vi "Check VIs for Dynamic Call Compatibility.vi"(8 "error in (no error)":errorcluster, 10 "VI 2":path, 11 "VI 1":path) -> (0 "error out":errorcluster, 3 "Compatible for dynamic call?":bool)   [LabVIEW 2017]
doc: "Given two VI paths, determine if those VIs have compatible connector panes for a dynamic call via a Call By Reference function. Note that this VI inspects the VI connector panes stored in the .vi files on disk, so this VI will not require loading the two VIs into memory. If the VIs are in memory, however, any changes to their connector panes will not be accurately reflected by this VI until those VIs are saved to disk."
uses:
  <vilib>/Utility/VariantDataType/VariantType.lvlib
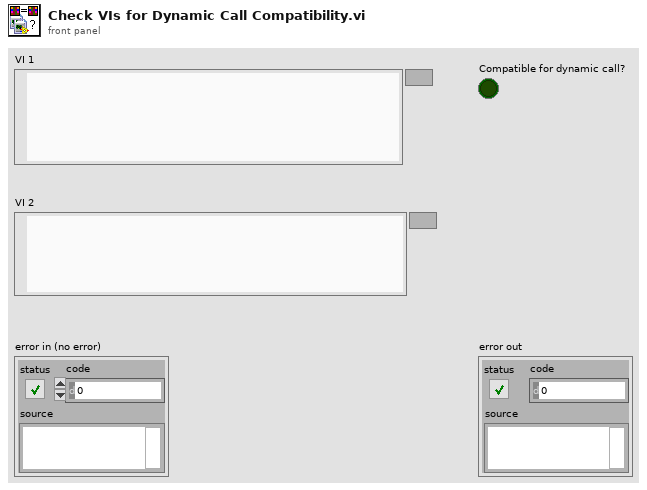
[diagram p1: front panel]
types:
  T1 = typedef "VariantType.lvlib/VIInfo.ctl" = cluster{"Data1":i16, "Data2":i16, "Flags":u32[], "Modification Date":timestamp, "Asynchronous":bool, "NonFunctional":bool, "Subroutine":bool, "SubSystem":bool}
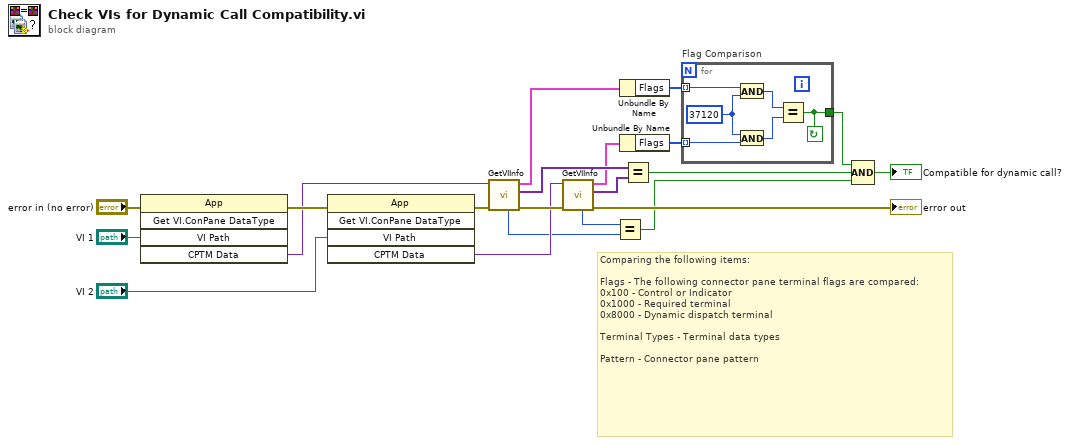
[diagram p0: block diagram]
diagram:
  # "Comparing the following items:\n\nFlags - The following connector pane terminal flags are compared:\n0x100 - Control or Indicator\n0x1000 - Required terminal\n0x8000 - Dynamic dispatch terminal\n\nTerminal Types - Terminal data types\n\nPattern - Connector pane pattern"
  n1 = invoke class="App" method="Get VI.ConPane DataType"(error in="error in (no error)", "VI Path"="VI 1") -> (error out=w21:errorcluster, "CPTM Data"=w17:variant)  [unwired: 3 in, 3 out]
  n2 = invoke class="App" method="Get VI.ConPane DataType"(error in=w21, "VI Path"="VI 2") -> (error out=w15:errorcluster, "CPTM Data"=w16:variant)  [unwired: 3 in, 3 out]
  n3 = call <vilib>:"GetVIInfo.vi"("error in (no error)"=w15, "Variant"=w17) -> ("error out"=w18:errorcluster, "VI Terminal Types"=w14:variant[], "VI Info"=w6:T1, "pattern"=w11:i16)  [unwired: 5 in, 1 out]
  n4 = call <vilib>:"GetVIInfo.vi"("error in (no error)"=w18, "Variant"=w16) -> ("error out"=→"error out":errorcluster, "VI Terminal Types"=w13:variant[], "VI Info"=w5:T1, "pattern"=w10:i16)  [unwired: 5 in, 1 out]
  n5 = Equal?(x=w10, y=w11) -> (x = y?=w7:bool)
  n6 = Unbundle By Name(w6) -> ("Flags"=w4:u32[])
  n7 = Unbundle By Name(w5) -> ("Flags"=w3:u32[])
  n8 = Equal?(x=w14, y=w13) -> (x = y?=w9:bool)
  n9 = for "Flag Comparison" {
    tunnel: w4 -> [w26] mode=indexing
    tunnel: w3 -> [w27] mode=indexing
    tunnel: [w23] -> w2
    stop <- w23 continue-if-true
    w22 = u32 37120 ("y")
    n10 = And(x=w26, y=w22) -> (x .and. y?=w25:u32)
    n11 = And(x=w22, y=w27) -> (x .and. y?=w24:u32)
    n12 = Equal?(x=w25, y=w24) -> (x = y?=w23:bool)
  }
  n13 = Compound Arithmetic op=AND(w2, w9, w7) -> (→"Compatible for dynamic call?":bool)
